vi "StopCore.vi"(6 "Timeout (ms)":i32=-1, 8 "error in (no error)":errorcluster, 11 "MicronGRPCClient in":refnum<class "MicronGRPCClient.lvclass">) -> (0 "error out":errorcluster, 2 "Response":string, 3 "MicronGRPCClient out":refnum<class "MicronGRPCClient.lvclass">)   [LabVIEW 2019, in "MicronGRPCClient.lvclass"]
uses:
  MicronGRPCClient.lvclass
  MicronGRPCClient.lvclass/MicronGRPCClient.ctl
  Base/Client/MicronClient.lvclass
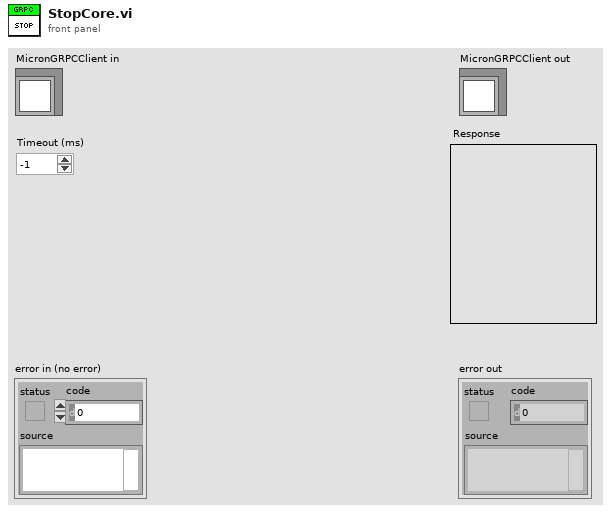
[diagram p1: front panel]
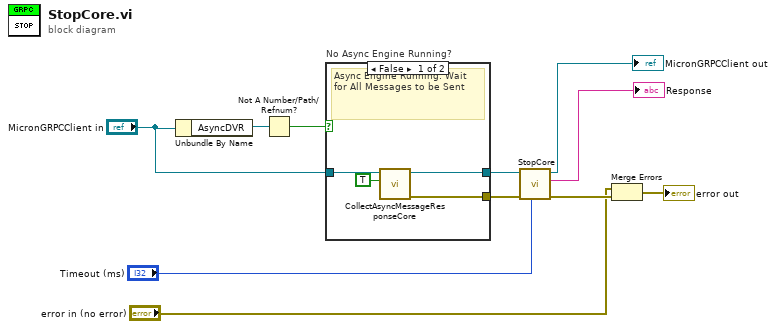
[diagram p0: block diagram]
diagram:
  n1 = Unbundle By Name("MicronGRPCClient in") -> ("AsyncDVR"=w7:refnum<data-value>)
  n2 = Not A Number/Path/Refnum?(number/path/refnum=w7) -> (NaN/Path/Refnum?=w3:bool)
  n3 = case "No Async Engine Running?" shown="False" w3 {
    tunnel: [w15 _] -> w6
    tunnel: "MicronGRPCClient in" -> [w14 w16]
    tunnel: [w13 w16] -> w4
    frame False {
      # "Async Engine Running. Wait for All Messages to be Sent"
      n4 = call-dynamic "CollectAsyncMessageResponseCore.vi"("Wait for All Messages?"=TRUE, "MicronGRPCClient in"=w14) -> ("error out"=w15:errorcluster, "MicronGRPCClient out"=w13:refnum<class "MicronGRPCClient.lvclass">)  [unwired: 7 in, 1 out]
    }
    frame True {
    }
  }
  n5 = call-parent "StopCore.vi"("Timeout (ms)"="Timeout (ms)", "error in (no error)"=w6, "MicronClient in"=w4) -> ("error out"=w11:errorcluster, "Response"=→"Response":string, "MicronClient out"=→"MicronGRPCClient out":refnum<class "MicronGRPCClient.lvclass">)  [unwired: 6 in]
  n6 = Merge Errors("error in (no error)", w11) -> (→"error out":errorcluster)
